vi "Interface.vi"() -> ()   [LabVIEW 2012]
uses:
  Control 1.ctl
panel:
  out "error out 2":errorcluster caption="error out"
  out "Frequency":dbl
  out "Period":dbl
  out "Duration":dbl
  out "Duty Cycle":dbl
  out "Preshoot":dbl
  out "Overshoot":dbl
  out "Slew Rate":dbl
  in  "Reset":bool
  in  "Capture":bool
  in  "X .10":bool
  in  "X10":bool
  in  "Position":dbl(knob) scale=-0.1..0.1 scale format="%#_2p"
  in  "Position":dbl(knob) scale=-10.0..10.0
  in  "Volts/Div":dbl(knob) scale=0.01..1.0 scale format="%#_6p"
  in  "GUI\nThreshold":dbl(knob)=2.5416638759420263 scale=-12.0..12.0
  in  "Reference":enum32{"AREF", "AVCC", "Reserved", "Internal"}(radio)
  in  "Trigger":enum32{"NGT", "PGT"}(radio)=enum."PGT"
  out "Graphical Representation of Data":T1
  out "Feedback \nfor shift\nregister":T2={"Threshold"=40, "Wait"=255, "Prescaler"=255, "Trigger"=130, "Vref"=255}
  out "Control Feedback Buffer":string
  out "Presets":string="Buffer size: 1280\r\nBaud rate: 115200\r\nWait duration: 1248\r\nPrescaler: 128\r\nTrigger event: 3\r\nThreshold: 127\r\n"
  out "error out":errorcluster
  in  "stop":bool
  in  "Seconds/Div":i32(knob)=4 min=1 max=7 step=1 scale=1.0..7.0 scale format="%.0p"
  in  "Intrument\nThreshold":i32(knob)=38 step=1 scale=0.0..255.0
  # "Voltage"
  # "Time"
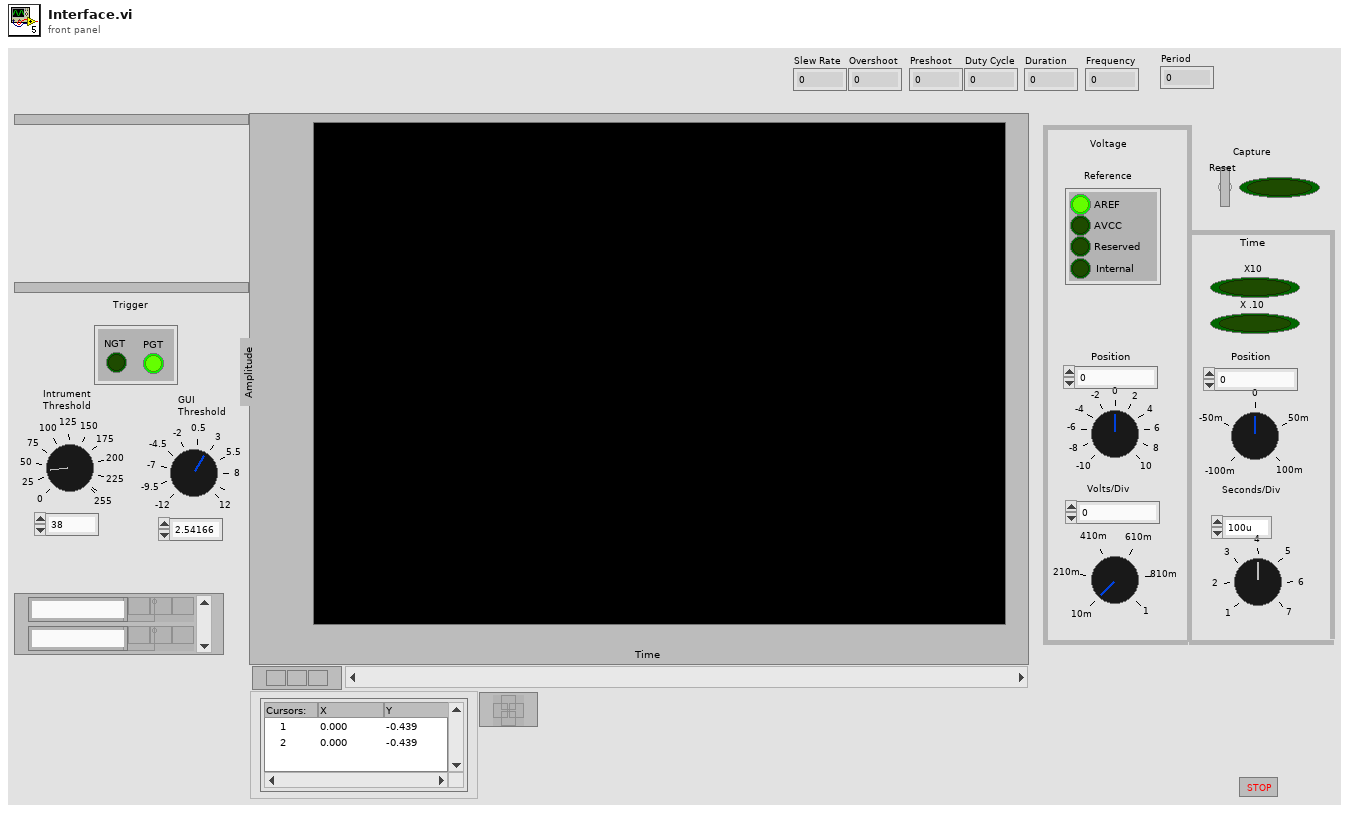
[diagram p1: front panel]
types:
  T1 = typedef "Control 1.ctl" = u8[]
  T2 = cluster{"Threshold":i32, "Wait":i32, "Prescaler":i32, "Trigger":i32, "Vref":i32}
  T3 = cluster{"f out":i32, "f out":i32, "Prescaler":i32, "Wait":i32, "f out":i32}
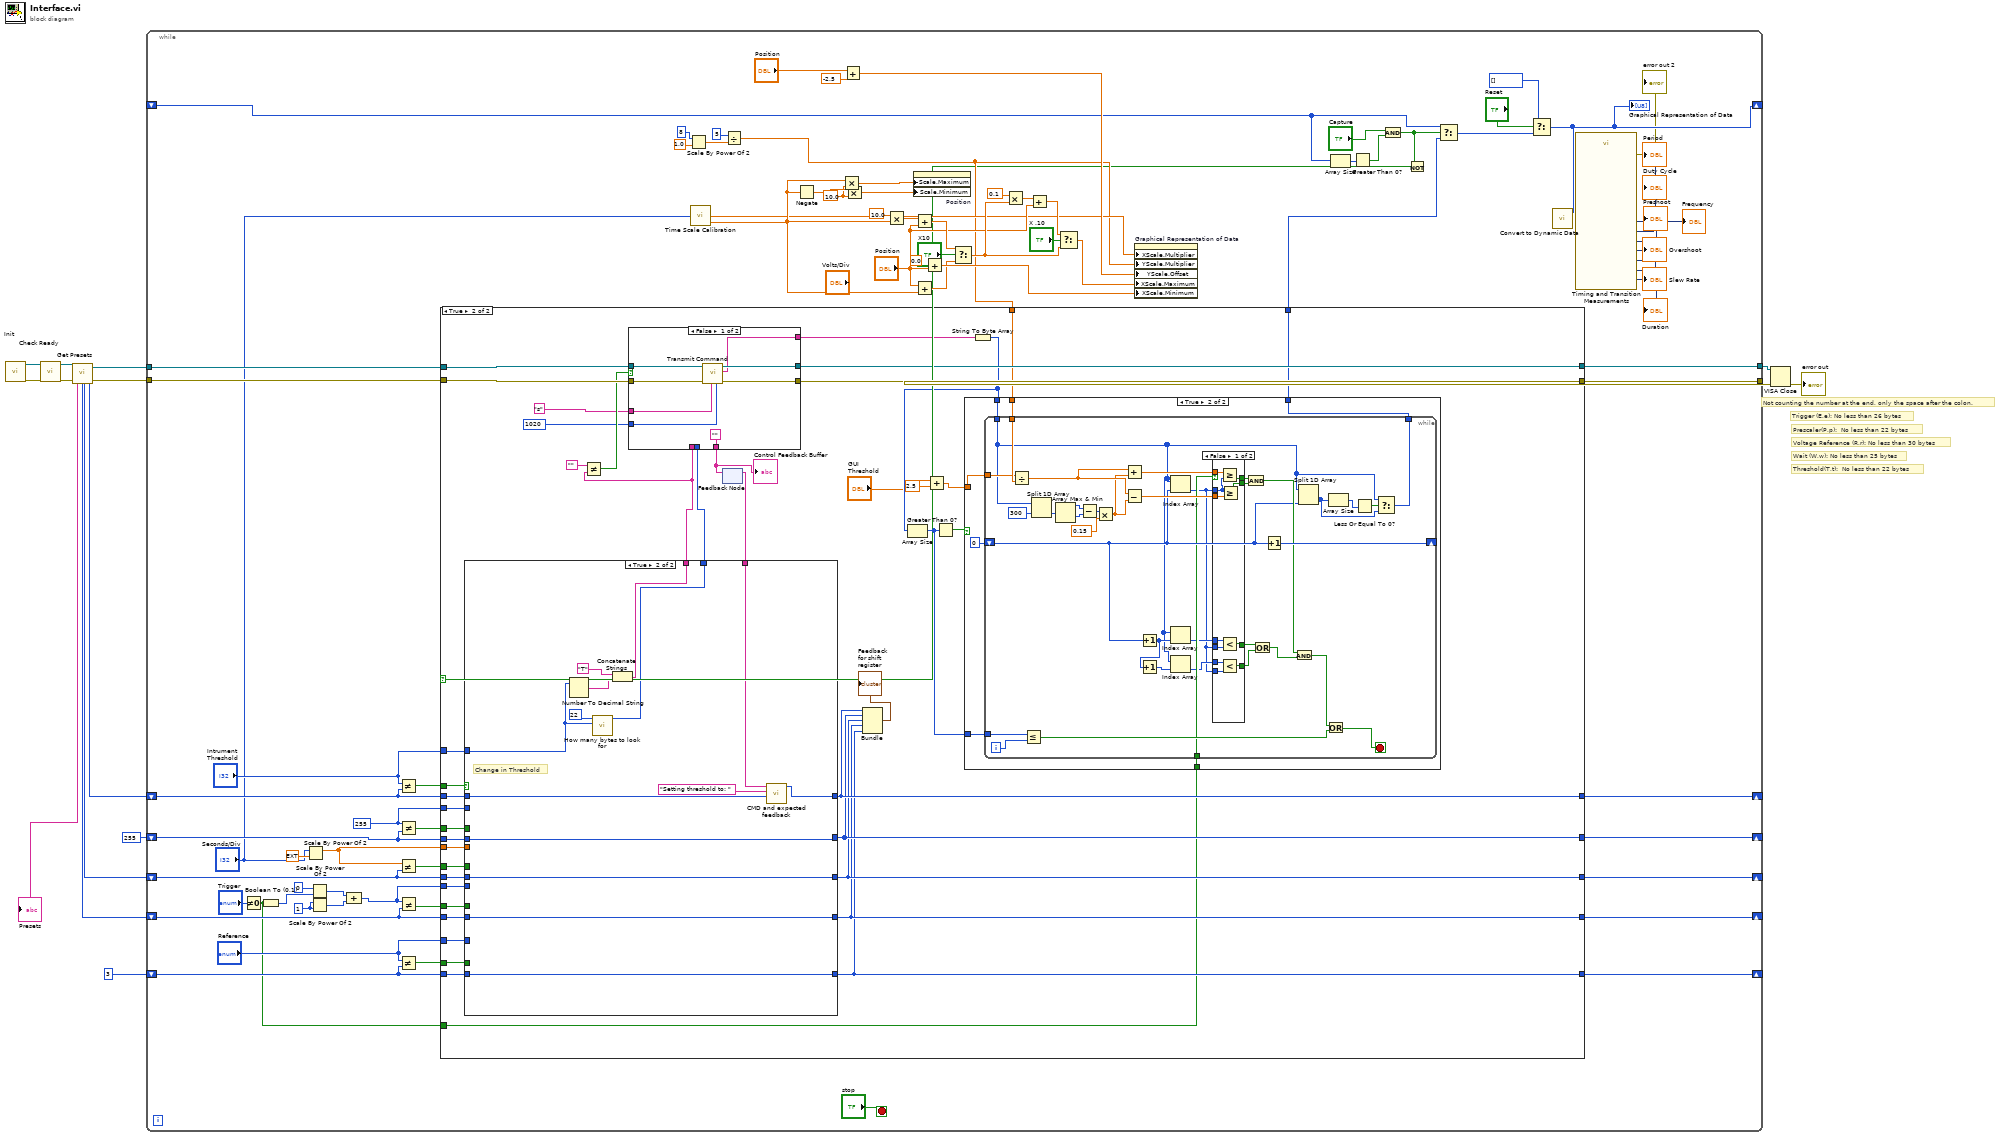
[diagram p0: block diagram]
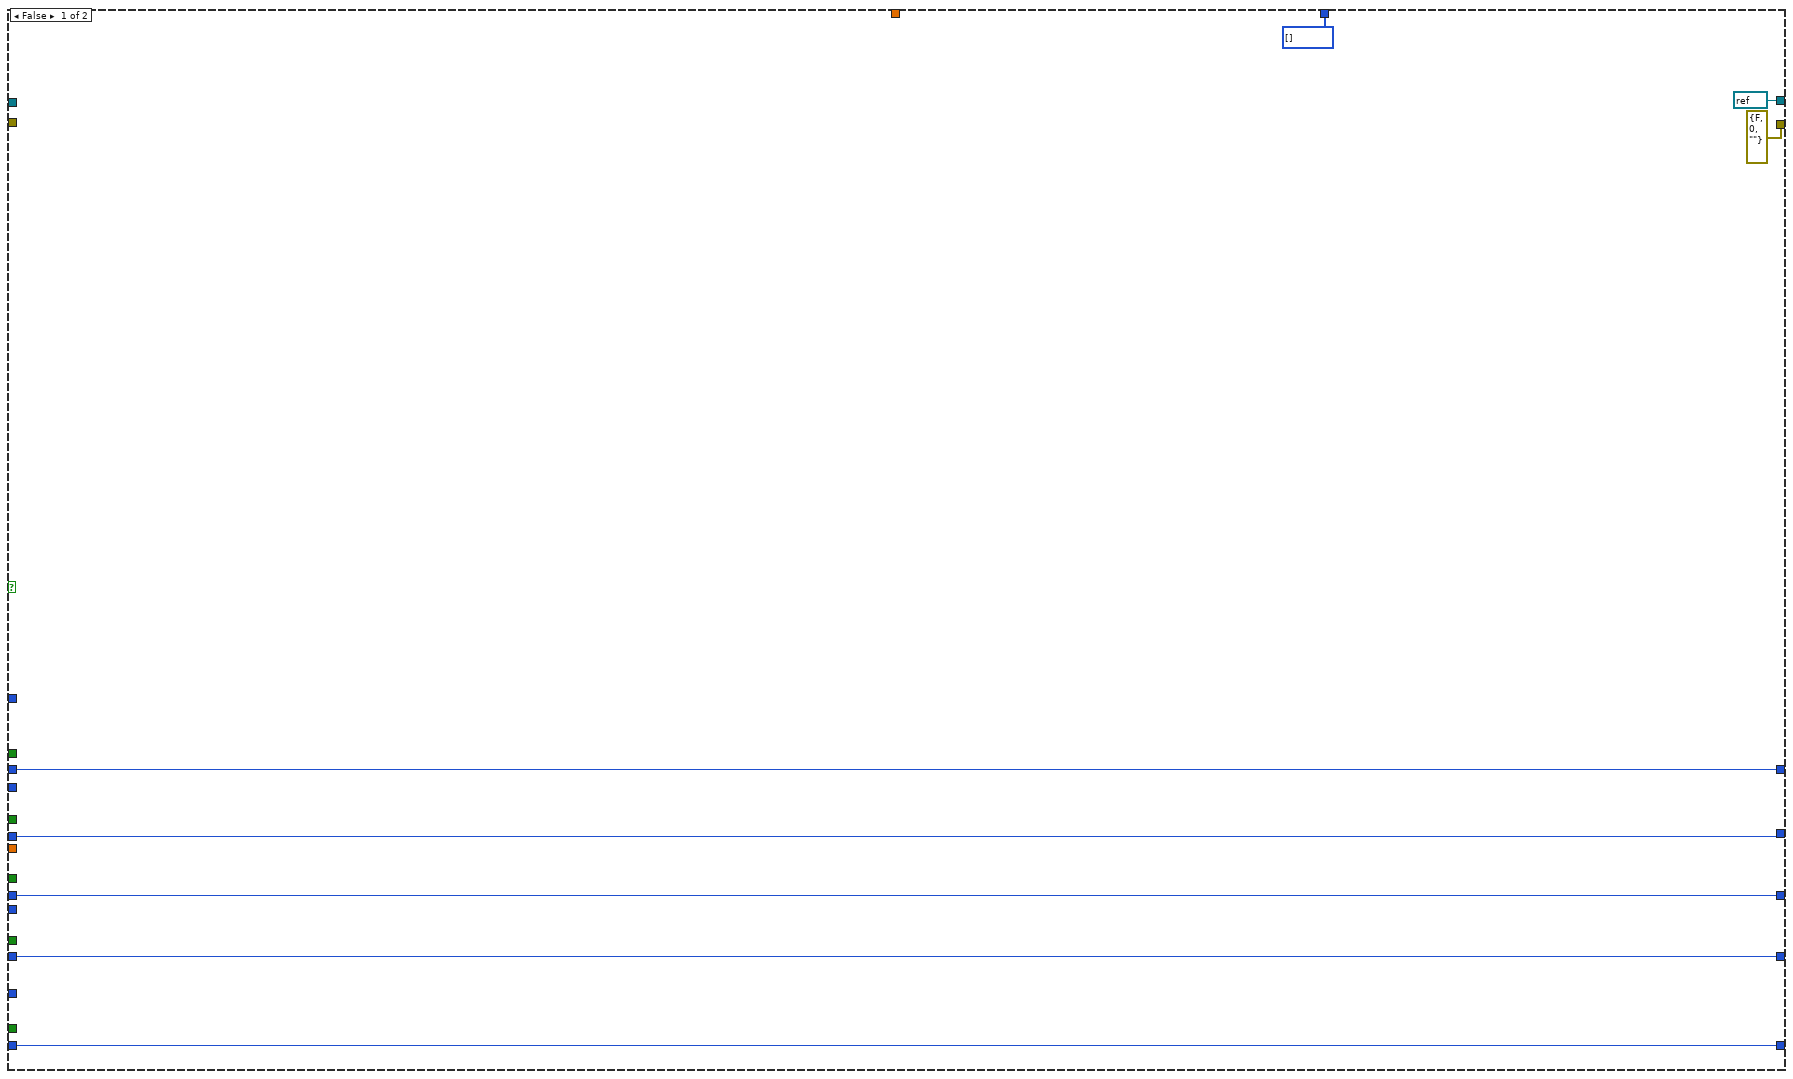
[diagram p2: hidden frame]
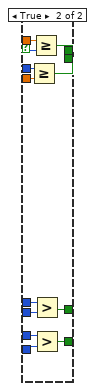
[diagram p4: hidden frame]
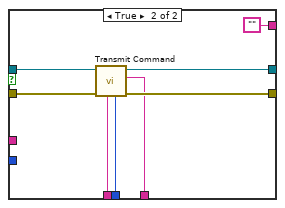
[diagram p5: hidden frame]
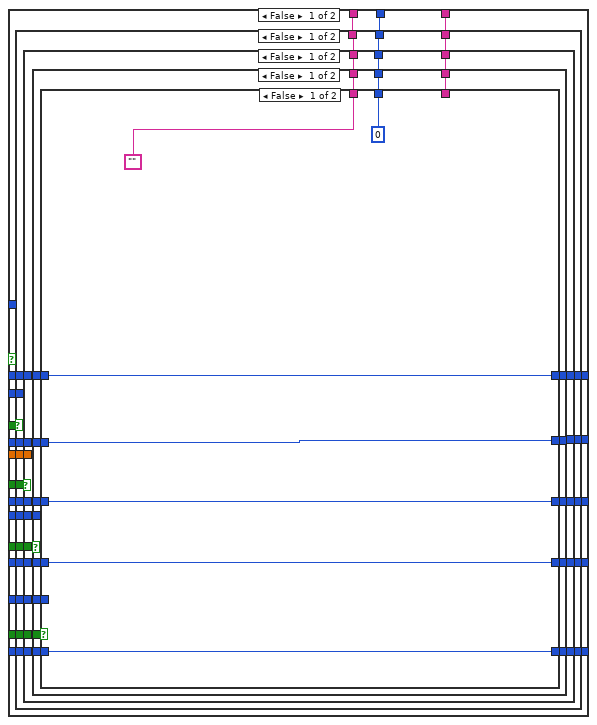
[diagram p6: hidden frame]
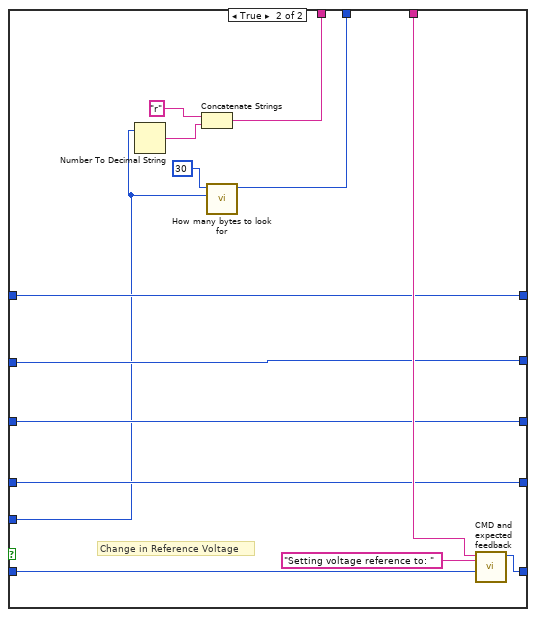
[diagram p7: hidden frame]
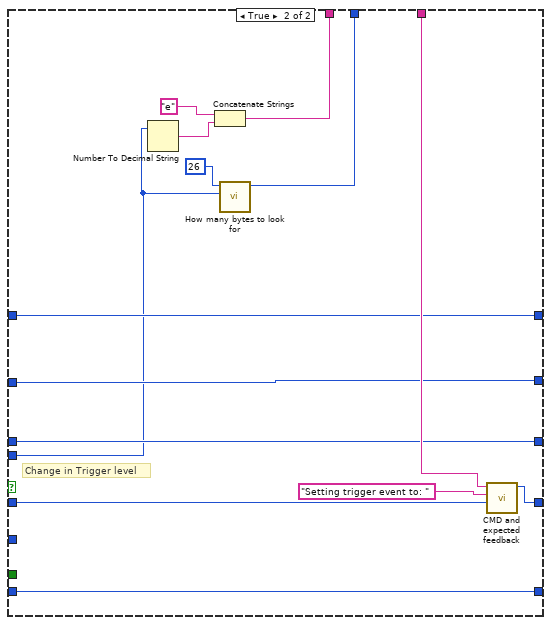
[diagram p8: hidden frame]
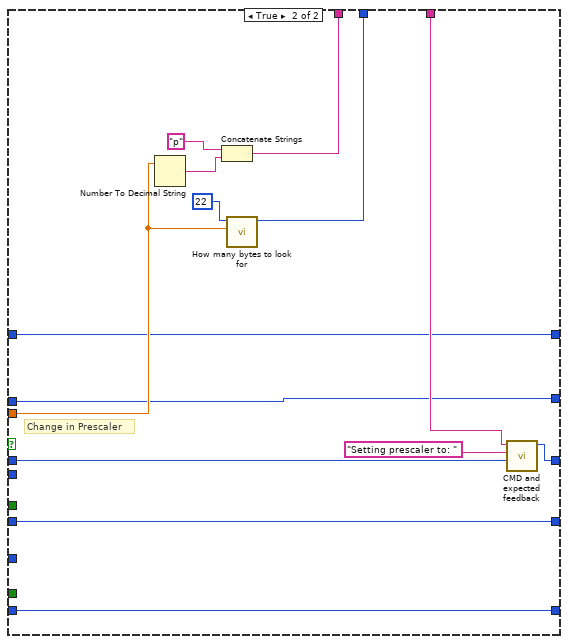
[diagram p9: hidden frame]
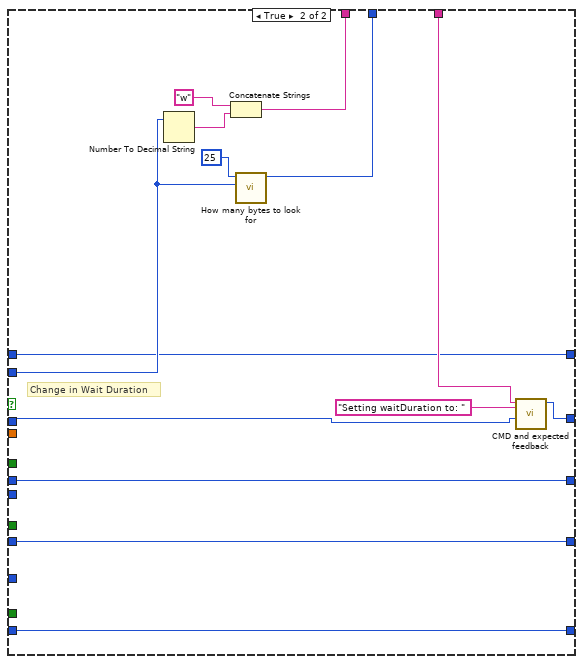
[diagram p10: hidden frame]
diagram:
  # "Not counting the number at the end, only the space after the colon."
  # "Prescaler(P,p):  No less than 22 bytes"
  # "Threshold(T,t):  No less than 22 bytes"
  # "Wait (W,w): No less than 25 bytes"
  # "Trigger (E,e): No less than 26 bytes"
  # "Voltage Reference (R,r): No less than 30 bytes"
  n1 = call "Init.vi"() -> ("error out"=w11:errorcluster, "VISA Refnum out"=w12:refnum<visa-resource-name>)  [unwired: 10 in]
  n2 = call "Check Ready.vi"("error in (no error)"=w11, "VISA Refnum in"=w12) -> ("error out"=w10:errorcluster, "VISA Refnum out"=w9:refnum<visa-resource-name>)  [unwired: 8 in]
  n3 = call "Get Presets.vi"("VISA Refnum in"=w9, "error in (no error)"=w10) -> ("read buffer"=→"Presets":string, "Wait"=w6:i32, "Prescaler"=w7:i32, "Threshold"=w4:i32, "VISA Refnum out"=w14:refnum<visa-resource-name>, "error out"=w13:errorcluster)  [unwired: 19 in, 1 out]
  n4 = while {
    tunnel: w13 -> [w84]
    tunnel: w14 -> [w85]
    shift-right: [w80] -> _
    shift-left: w4 -> [w86]
    shift-right: [w79] -> _
    shift-left: 255 ("f out") -> [w81]
    shift-right: [w78] -> _
    shift-left: w7 -> [w87]
    shift-right: [w77] -> _
    shift-left: w6 -> [w88]
    shift-right: [w76] -> _
    shift-left: 3 -> [w89]
    tunnel: [w83] -> w3
    tunnel: [w82] -> w2
    shift-right: [w25] -> _
    shift-left: _ -> [w33]
    stop <- "stop" stop-if-true
    w26 = 10.0 ("y")
    w90 = 255 ("Wait")
    w74 = 1 ("x")
    n5 = Not Equal To 0?(x="Trigger") -> (x != 0?=w39:bool)
    n6 = Boolean To (0,1)(Boolean=w39) -> (0, 1=w70:i16)
    n7 = Scale By Power Of 2(n="Seconds/Div", x=ext 1.0) -> (x*2^n=w63:ext)
    n8 = Scale By Power Of 2(n=0, x=w70) -> (x*2^n=w69:i16)
    n9 = Scale By Power Of 2(n=w74, x=w74) -> (x*2^n=w73:i32)
    n10 = Compound Arithmetic op=unknown(w69, w73) -> (w72:i32)
    n11 = Not Equal?(x="Intrument\nThreshold", y=w86) -> (x != y?=w96:bool)
    n12 = Not Equal?(x=w63, y=w87) -> (x != y?=w93:bool)
    n13 = Not Equal?(x="Reference", y=w89) -> (x != y?=w95:bool)
    n14 = Not Equal?(x=w90, y=w81) -> (x != y?=w92:bool)
    n15 = Not Equal?(x=w72, y=w88) -> (x != y?=w94:bool)
    n16 = Scale By Power Of 2(n=i16 8, x=1.0) -> (x*2^n=w64:dbl)
    n17 = call "Time Scale Calibration.vi"("Numeric"="Seconds/Div") -> ("max time"=w52:dbl, "Time Scale Multiplier"=w41:dbl)  [unwired: 3 in]
    n18 = Divide(x=5, y=w64) -> (x/y=w40:dbl)
    n19 = Negate(x=w52) -> (-x=w54:dbl)
    n20 = Multiply(x=w52, y=w26) -> (x*y=w28:dbl)
    n21 = Add(x="Position", y=-2.5 ("Y Scale.Offset and Multiplier:Offset")) -> (x+y=w59:dbl)
    n22 = Multiply(x=w54, y=w26) -> (x*y=w27:dbl)
    n23 = Multiply(x=10.0, y=w52) -> (x*y=w50:dbl)
    n24 = property on="Position" class="Knob (strict)"("Scale.Maximum"=w28, "Scale.Minimum"=w27) -> ()  [unwired: 2 in, 2 out]
    n25 = Add(x=w50, y="Position") -> (x+y=w49:dbl)
    n26 = Add(x="Position", y=w52) -> (x+y=w55:dbl)
    n27 = Add(x=0.0 ("X Scale.Range:Minimum"), y="Position") -> (x+y=w57:dbl)
    n28 = Select(t=w49, s="X10", f=w55) -> (s? t:f=w43:dbl)
    n29 = Multiply(x=0.1, y=w43) -> (x*y=w46:dbl)
    n30 = Add(x=w46, y="Position") -> (x+y=w45:dbl)
    n31 = Select(t=w45, s="X .10", f=w43) -> (s? t:f=w48:dbl)
    n32 = property on="Graphical Representation of Data" class="WFGraph (strict)"("XScale.Multiplier"=w41, "YScale.Multiplier"=w40, "YScale.Offset"=w59, "XScale.Maximum"=w48, "XScale.Minimum"=w57) -> ()  [unwired: 2 in, 2 out]
    n33 = Array Size(array=w33) -> (size(s)=w35:i32)
    n34 = Greater Than 0?(x=w35) -> (x > 0?=w34:bool)
    n35 = And(x="Capture", y=w34) -> (x .and. y?=w30:bool)
    n36 = Not(x=w30) -> (.not. x?=w29:bool)
    n37 = case shown="True" w29 {
      tunnel: w96 -> [_ w148]
      tunnel: w95 -> [_ w147]
      tunnel: w94 -> [_ w146]
      tunnel: w93 -> [_ w145]
      tunnel: w92 -> [_ w144]
      tunnel: "Intrument\nThreshold" -> [_ w143]
      tunnel: w90 -> [_ w142]
      tunnel: w89 -> [w98 w141]
      tunnel: w88 -> [w99 w140]
      tunnel: w87 -> [w100 w139]
      tunnel: w86 -> [w102 w138]
      tunnel: w85 -> [_ w137]
      tunnel: w84 -> [_ w136]
      tunnel: [refnum<visa-resource-name> refnum ("VISA Refnum out") w134] -> w83
      tunnel: [errorcluster {"status"=FALSE, "code"=0, "source"=""} ("error out") w133] -> w82
      tunnel: w81 -> [w101 w131]
      tunnel: [w102 w129] -> w80
      tunnel: [w101 w128] -> w79
      tunnel: [w100 w127] -> w78
      tunnel: [w99 w126] -> w77
      tunnel: [w98 w125] -> w76
      tunnel: w72 -> [_ w118]
      tunnel: "Reference" -> [_ w117]
      tunnel: w63 -> [_ w109]
      tunnel: w40 -> [_ w108]
      tunnel: w39 -> [_ w107]
      tunnel: [u8[] [] ("unsigned byte array") w106] -> w32
      frame False {
      }
      frame True {
        n38 = feedback #1() -> (w132:string)  [unwired: 1 in]
        n39 = case shown="True" w148 {
          tunnel: w147 -> [w251 _]
          tunnel: w146 -> [w250 _]
          tunnel: w145 -> [w249 _]
          tunnel: w144 -> [w248 _]
          tunnel: w143 -> [_ w377]
          tunnel: w142 -> [w245 _]
          tunnel: w109 -> [w243 _]
          tunnel: w118 -> [w235 _]
          tunnel: w117 -> [w236 _]
          tunnel: w141 -> [w240 w366]
          tunnel: w140 -> [w241 w367]
          tunnel: w139 -> [w242 w368]
          tunnel: w138 -> [w239 w371]
          tunnel: [w246 w375] -> w135
          tunnel: [w247 w374] -> w123
          tunnel: w132 -> [w244 w373]
          tunnel: [w232 w370] -> w129
          tunnel: w131 -> [w233 w369]
          tunnel: [w238 w369] -> w128
          tunnel: [w237 w367] -> w126
          tunnel: [w234 w366] -> w125
          tunnel: [w231 w368] -> w127
          frame False {
            n40 = case shown="False" w248 {
              tunnel: w251 -> [w270 _]
              tunnel: w250 -> [w269 _]
              tunnel: w249 -> [w268 _]
              tunnel: [w265 w362] -> w247
              tunnel: [w266 w361] -> w246
              tunnel: w245 -> [_ w360]
              tunnel: w244 -> [w267 w359]
              tunnel: w243 -> [w264 _]
              tunnel: w242 -> [w263 w356]
              tunnel: w241 -> [w262 w354]
              tunnel: w240 -> [w260 w353]
              tunnel: w239 -> [w261 w355]
              tunnel: [w254 w357] -> w238
              tunnel: [w259 w354] -> w237
              tunnel: w236 -> [w258 _]
              tunnel: w235 -> [w257 _]
              tunnel: [w256 w353] -> w234
              tunnel: w233 -> [w255 w352]
              tunnel: [w253 w355] -> w232
              tunnel: [w252 w356] -> w231
              frame False {
                n41 = case shown="False" w268 {
                  tunnel: w270 -> [w287 _]
                  tunnel: w269 -> [w286 _]
                  tunnel: w267 -> [w285 w348]
                  tunnel: [w271 w347] -> w266
                  tunnel: [w272 w346] -> w265
                  tunnel: w264 -> [_ w345]
                  tunnel: w263 -> [w281 w343]
                  tunnel: w262 -> [w284 w340]
                  tunnel: w261 -> [w283 w342]
                  tunnel: w260 -> [w280 w339]
                  tunnel: [w282 w340] -> w259
                  tunnel: w258 -> [w279 _]
                  tunnel: w257 -> [w278 _]
                  tunnel: [w277 w339] -> w256
                  tunnel: w255 -> [w276 w341]
                  tunnel: [w275 w341] -> w254
                  tunnel: [w274 w342] -> w253
                  tunnel: [w273 w338] -> w252
                  frame False {
                    n42 = case shown="False" w286 {
                      tunnel: w287 -> [w302 _]
                      tunnel: w285 -> [w301 w336]
                      tunnel: w284 -> [w300 w337]
                      tunnel: w283 -> [w299 w333]
                      tunnel: [w294 w334] -> w282
                      tunnel: w281 -> [w298 w330]
                      tunnel: w280 -> [w297 w331]
                      tunnel: w279 -> [w296 _]
                      tunnel: w278 -> [_ w324]
                      tunnel: [w295 w331] -> w277
                      tunnel: w276 -> [w293 w332]
                      tunnel: [w292 w332] -> w275
                      tunnel: [w291 w333] -> w274
                      tunnel: [w290 w330] -> w273
                      tunnel: [w289 w326] -> w272
                      tunnel: [w288 w325] -> w271
                      frame False {
                        n43 = case shown="False" w302 {
                          tunnel: w301 -> [_ w321]
                          tunnel: w300 -> [w307 w319]
                          tunnel: w299 -> [w309 w317]
                          tunnel: w298 -> [w305 w316]
                          tunnel: w297 -> [w306 w322]
                          tunnel: w296 -> [_ w311]
                          tunnel: [w306 w323] -> w295
                          tunnel: [w307 w319] -> w294
                          tunnel: w293 -> [w308 w318]
                          tunnel: [w308 w318] -> w292
                          tunnel: [w309 w317] -> w291
                          tunnel: [w305 w316] -> w290
                          tunnel: ["" w312] -> w289
                          tunnel: [i64 0 ("Numeric out") w310] -> w288
                          frame False {
                          }
                          frame True {
                            # "Change in Reference Voltage"
                            n44 = Number To Decimal String(number=w311) -> (decimal integer string=w315:string)  [unwired: 1 in]
                            n45 = Concatenate Strings("r" ("string"), w315) -> (w312:string)
                            n46 = call "How many bytes to look for.vi"("x"=w311, "Numeric in"=30) -> ("Numeric out"=w310:i64)  [unwired: 9 in]
                            n47 = call "CMD and expected feedback.vi"("f in"=w322, "y"="Setting voltage reference to: ", "string"=w321) -> ("f out"=w323:i32)  [unwired: 8 in]
                          }
                        }
                      }
                      frame True {
                        # "Change in Trigger level"
                        n48 = Number To Decimal String(number=w324) -> (decimal integer string=w329:string)  [unwired: 1 in]
                        n49 = Concatenate Strings("e" ("string"), w329) -> (w326:string)
                        n50 = call "How many bytes to look for.vi"("x"=w324, "Numeric in"=26) -> ("Numeric out"=w325:i64)  [unwired: 9 in]
                        n51 = call "CMD and expected feedback.vi"("f in"=w337, "y"="Setting trigger event to: ", "string"=w336) -> ("f out"=w334:i32)  [unwired: 8 in]
                      }
                    }
                  }
                  frame True {
                    # "Change in Prescaler"
                    n52 = Number To Decimal String(number=w345) -> (decimal integer string=w351:string)  [unwired: 1 in]
                    n53 = Concatenate Strings("p" ("string"), w351) -> (w346:string)
                    n54 = call "How many bytes to look for.vi"("x"=w345, "Numeric in"=22) -> ("Numeric out"=w347:i64)  [unwired: 9 in]
                    n55 = call "CMD and expected feedback.vi"("f in"=w343, "y"="Setting prescaler to: ", "string"=w348) -> ("f out"=w338:i32)  [unwired: 8 in]
                  }
                }
              }
              frame True {
                # "Change in Wait Duration"
                n56 = Number To Decimal String(number=w360) -> (decimal integer string=w365:string)  [unwired: 1 in]
                n57 = Concatenate Strings("w" ("string"), w365) -> (w362:string)
                n58 = call "How many bytes to look for.vi"("x"=w360, "Numeric in"=25) -> ("Numeric out"=w361:i64)  [unwired: 9 in]
                n59 = call "CMD and expected feedback.vi"("f in"=w352, "y"="Setting waitDuration to: ", "string"=w359) -> ("f out"=w357:i32)  [unwired: 8 in]
              }
            }
          }
          frame True {
            # "Change in Threshold"
            n60 = Number To Decimal String(number=w377) -> (decimal integer string=w379:string)  [unwired: 1 in]
            n61 = call "How many bytes to look for.vi"("x"=w377, "Numeric in"=22) -> ("Numeric out"=w375:i64)  [unwired: 9 in]
            n62 = Concatenate Strings("T" ("string"), w379) -> (w374:string)
            n63 = call "CMD and expected feedback.vi"("f in"=w371, "y"="Setting threshold to: ", "string"=w373) -> ("f out"=w370:i32)  [unwired: 8 in]
          }
        }
        n64 = Not Equal?(x="", y=w123) -> (x != y?=w121:bool)
        n65 = case shown="False" w121 {
          tunnel: w137 -> [w220 w230]
          tunnel: w136 -> [w221 w229]
          tunnel: w135 -> [_ w228]
          tunnel: [w219 w227] -> w134
          tunnel: [w218 w226] -> w133
          tunnel: ["" ("read buffer") w225] -> w130
          tunnel: w123 -> [_ w224]
          tunnel: 1020 ("CMD\nBytes  to look for") -> [w217 _]
          tunnel: "s" ("CMD") -> [w216 _]
          tunnel: [w215 "" ("read buffer")] -> w116
          frame False {
            n66 = call "Transmit Command.vi"("Numeric"=w217, "String"=w216, "error in (no error)"=w221, "VISA Refnum in"=w220) -> ("error out"=w218:errorcluster, "read buffer"=w215:string, "VISA Refnum out"=w219:refnum<visa-resource-name>)  [unwired: 5 in]
          }
          frame True {
            n67 = call "Transmit Command.vi"("Numeric"=w228, "String"=w224, "error in (no error)"=w229, "VISA Refnum in"=w230) -> ("error out"=w226:errorcluster, "read buffer"=w225:string, "VISA Refnum out"=w227:refnum<visa-resource-name>)  [unwired: 5 in]
          }
        }
        "Control Feedback Buffer" <- w130
        n68 = feedback-in #1(w130) -> ()
        n69 = Bundle("f out"=w129, "f out"=w128, "Prescaler"=w127, "Wait"=w126, "f out"=w125) -> (→"Feedback \nfor shift\nregister":T3)  [unwired: 1 in]
        n70 = Add(x="GUI\nThreshold", y=2.5) -> (x+y=w111:dbl)
        n71 = String To Byte Array(string=w116) -> (unsigned byte array=w114:u8[])
        n72 = Array Size(array=w114) -> (size(s)=w113:i32)
        n73 = Greater Than 0?(x=w113) -> (x > 0?=w115:bool)
        n74 = case shown="True" w115 {
          tunnel: w114 -> [w149 w156]
          tunnel: w108 -> [_ w155]
          tunnel: w111 -> [_ w154]
          tunnel: [w149 w152] -> w106
          tunnel: w113 -> [_ w151]
          tunnel: w107 -> [_ w150]
          frame False {
          }
          frame True {
            n75 = while {
              tunnel: w156 -> [w164]
              tunnel: w155 -> [w186]
              tunnel: w154 -> [w185]
              shift-right: [w182] -> _
              shift-left: 0 -> [w173]
              tunnel: [w163] -> w152
              tunnel: w151 -> [w171]
              tunnel: w150 -> [w162]
              i -> [w172]
              stop <- w168 stop-if-true
              n76 = Divide(x=w185, y=w186) -> (x/y=w184:dbl)
              n77 = Less Or Equal?(x=w171, y=w172) -> (x <= y?=w170:bool)
              n78 = Split 1D Array(array=w164, index=300) -> (second subarray=w191:u8[])  [unwired: 1 out]
              n79 = Array Max & Min(array=w191) -> (max value=w190:u8, min value=w189:u8)  [unwired: 2 out]
              n80 = Subtract(x=w190, y=w189) -> (x-y=w188:u8)
              n81 = Multiply(x=w188, y=0.15) -> (x*y=w183:dbl)
              n82 = Add(x=w184, y=w183) -> (x+y=w181:dbl)
              n83 = Subtract(x=w184, y=w183) -> (x-y=w180:dbl)
              n84 = Increment(x=w173) -> (x+1=w177:i32)
              n85 = Increment(x=w177) -> (x+1=w176:i32)
              n86 = Index Array(array=w164, index=w177) -> (element=w159:u8)
              n87 = Index Array(array=w164, index=w176) -> (element=w158:u8)
              n88 = Index Array(array=w164, index=w173) -> (element=w157:u8)
              n89 = case shown="False" w162 {
                tunnel: w181 -> [w201 w214]
                tunnel: w180 -> [w200 w213]
                tunnel: [w203 w212] -> w179
                tunnel: [w202 w211] -> w178
                tunnel: w157 -> [w199 w210]
                tunnel: [w196 w209] -> w161
                tunnel: [w197 w208] -> w160
                tunnel: w159 -> [w198 w207]
                tunnel: w158 -> [w195 w206]
                tunnel: w157 -> [w194 w205]
                tunnel: w157 -> [w193 w204]
                frame False {
                  n90 = Greater Or Equal?(x=w201, y=w199) -> (x >= y?=w203:bool)
                  n91 = Less?(x=w198, y=w193) -> (x < y?=w197:bool)
                  n92 = Less?(x=w195, y=w194) -> (x < y?=w196:bool)
                  n93 = Greater Or Equal?(x=w199, y=w200) -> (x >= y?=w202:bool)
                }
                frame True {
                  n94 = Greater Or Equal?(x=w210, y=w213) -> (x >= y?=w211:bool)
                  n95 = Greater Or Equal?(x=w214, y=w210) -> (x >= y?=w212:bool)
                  n96 = Greater?(x=w207, y=w204) -> (0:w208:bool)
                  n97 = Greater?(x=w206, y=w205) -> (0:w209:bool)
                }
              }
              n98 = And(x=w179, y=w178) -> (x .and. y?=w175:bool)
              n99 = Or(x=w160, y=w161) -> (x .or. y?=w174:bool)
              n100 = Increment(x=w173) -> (x+1=w182:i32)
              n101 = And(x=w175, y=w174) -> (x .and. y?=w169:bool)
              n102 = Split 1D Array(array=w164, index=w173) -> (second subarray=w165:u8[])  [unwired: 1 out]
              n103 = Or(x=w169, y=w170) -> (x .or. y?=w168:bool)
              n104 = Array Size(array=w165) -> (size(s)=w167:i32)
              n105 = Less Or Equal To 0?(x=w167) -> (x <= 0?=w166:bool)
              n106 = Select(t=w164, s=w166, f=w165) -> (s? t:f=w163:u8[])
            }
          }
        }
      }
    }
    n107 = Select(t=w33, s=w30, f=w32) -> (s? t:f=w37:u8[])
    n108 = Select(t=u8[] [], s="Reset", f=w37) -> (s? t:f=w25:u8[])
    "Graphical Representation of Data" <- w25
    n109 = call "Convert to Dynamic Data"("Array"=w25) -> ("Dynamic Data Type"=w24:dynamicdata)  [unwired: 3 in]
    n110 = call "Timing and Transition Measurements"("Signals"=w24) -> ("error out"=→"error out 2":errorcluster, "Frequency"=→"Frequency":dynamicdata, "Period"=→"Period":dynamicdata, "Duration"=→"Duration":dynamicdata, "Duty Cycle"=→"Duty Cycle":dynamicdata, "Preshoot"=→"Preshoot":dynamicdata, "Overshoot"=→"Overshoot":dynamicdata, "Slew Rate"=→"Slew Rate":dynamicdata)  [unwired: 3 in]
  }
  n111 = VISA Close(VISA resource name=w3, error in (no error)=w2) -> (error out=→"error out":errorcluster)
